vi "PopulateSupportedBinning.vi"(10 "Binning":refnum<vi>, 11 ".NET Refnum in":refnum<k24>) -> ()   [LabVIEW 2019]
uses:
  Dependencies/PVCamNET.dll
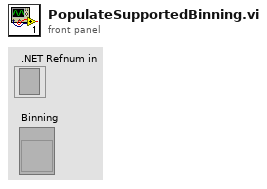
[diagram p1: front panel]
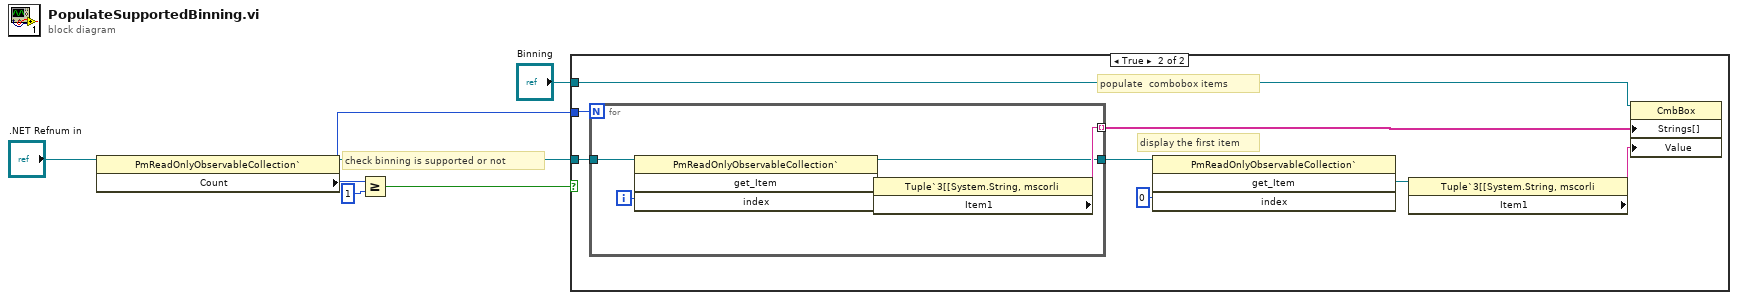
[diagram p0: block diagram]
diagram:
  # "check binning is supported or not"
  n1 = property class="PmReadOnlyObservableCollection`"(reference=".NET Refnum in") -> (reference out=w2:refnum<k24>, "Count"=w4:i32)  [unwired: 1 in, 1 out]
  n2 = Greater Or Equal?(x=w4, y=u16 1) -> (x >= y?=w5:bool)
  n3 = case shown="True" w5 {
    tunnel: w2 -> [_ w14]
    tunnel: w4 -> [_ w8]
    tunnel: "Binning" -> [_ w7]
    frame False {
    }
    frame True {
      # "display the first item"
      # "populate  combobox items"
      n4 = for {
        N: w8 -> [_]
        tunnel: w14 -> [w19]
        tunnel: [w16] -> w13 mode=indexing
        tunnel: [w15] -> w12
        i -> [w18]
        n5 = invoke class="PmReadOnlyObservableCollection`" method="get_Item"(reference=w19, "index"=w18) -> (reference out=w15:refnum<k24>, "get_Item"=w17:refnum<k24>)  [unwired: 2 in, 2 out]
        n6 = property class="Tuple`3[[System.String, mscorli"(reference=w17) -> ("Item1"=w16:string)  [unwired: 1 in, 2 out]
      }
      n7 = invoke class="PmReadOnlyObservableCollection`" method="get_Item"(reference=w12, "index"=0) -> ("get_Item"=w10:refnum<k24>)  [unwired: 2 in, 3 out]
      n8 = property class="Tuple`3[[System.String, mscorli"(reference=w10) -> ("Item1"=w9:string)  [unwired: 1 in, 2 out]
      n9 = property class="CmbBox"(reference=w7, "Strings[]"=w13, "Value"=w9) -> ()  [unwired: 1 in, 2 out]
    }
  }
